vi "Practica1.1_Graficos.vi"() -> ()   [LabVIEW 2022 SP3]
uses:
  <vilib>/measure/NI_MABase.lvlib
panel:
  in  "Amplitud":dbl(slide) scale=0.0..10.0
  in  "Control de velocidad":dbl(knob) scale=0.0..10.0
  out "Waveform Graph":waveform(dbl)(graph)
  out "Waveform Chart":dbl(graph)
  # "Anahí Montserrat Vázquez Padilla \nPráctica 03:Gráficos\n30/01/2024"
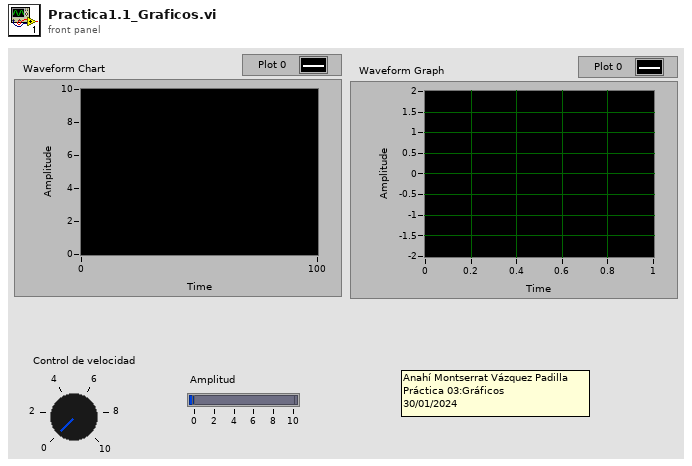
[diagram p1: front panel]
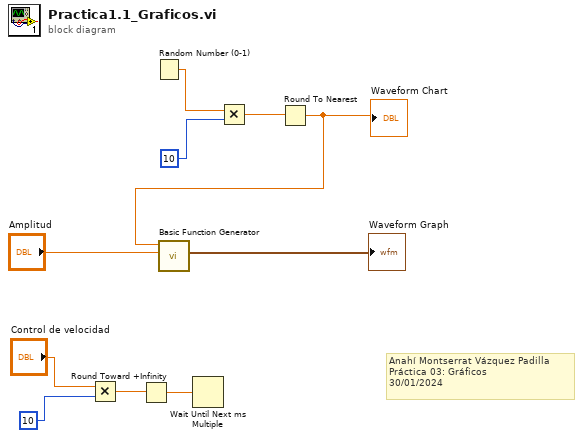
[diagram p0: block diagram]
diagram:
  # "Anahí Montserrat Vázquez Padilla \nPráctica 03: Gráficos \n30/01/2024"
  n1 = Multiply(x="Control de velocidad", y=10) -> (x*y=w2:dbl)
  n2 = Round Toward +Infinity(x=w2) -> (ceil(x): smallest int >= x=w1:dbl)
  n3 = Random Number (0-1)() -> (number: 0 to 1=w10:dbl)
  n4 = Wait Until Next ms Multiple(millisecond multiple=w1) -> ()  [unwired: 1 out]
  n5 = Multiply(x=w10, y=10) -> (x*y=w8:dbl)
  n6 = Round To Nearest(number=w8) -> (nearest integer value=w6:dbl)
  "Waveform Chart" <- w6
  n7 = call <vilib>:"Basic Function Generator.vi"("amplitude"="Amplitud", "frequency"=w6) -> ("signal out"=→"Waveform Graph":waveform(dbl))  [unwired: 7 in, 2 out]
